vi "create client connector.vi"(8 "error in":errorcluster, 11 "engine":u64) -> (0 "error out":errorcluster, 3 "client out":u64)   [LabVIEW 2016, in "async tls.lvlib"]
uses:
  async tls.lvlib
  lvasynctls.dll
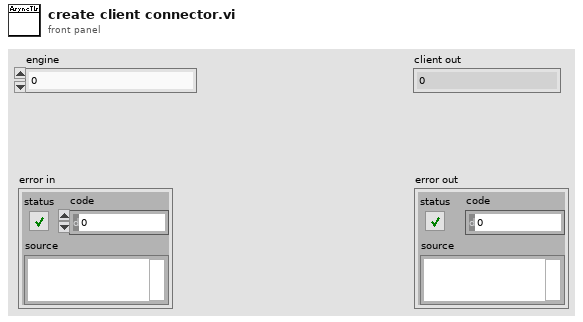
[diagram p1: front panel]
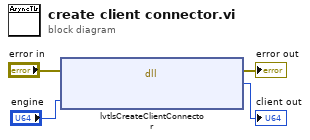
[diagram p0: block diagram]
diagram:
  n1 = dll-call lib="C:/Users/IEUser/Desktop/libasynclvtls/lvasynctls.dll" fn="lvtlsCreateClientConnector"(error in="error in", "engine"="engine") -> (error out=→"error out":errorcluster, "client"=→"client out":u64)  [unwired: 3 in, 1 out]
